vi "Initialize.vi"(5 "Replication Offset":dbl, 7 "Flip Rotation?":bool, 8 "error in (no error)":errorcluster, 9 "Spawner Early Search":T1, 10 "Initial Direction Offset":T1, 11 "Test in":refnum<class "Swarm.lvclass">) -> (0 "error out":errorcluster, 3 "Test out":refnum<class "Swarm.lvclass">)   [LabVIEW 2020, in "Swarm.lvclass"]
uses:
  Swarm.lvclass
  Type Defs/Direction Enum.ctl
  Type Defs/Action Enum.ctl
  Swarm.lvclass/Swarm.ctl
  Type Defs/SB Type Defs.lvlib
  Common/Common.lvlib
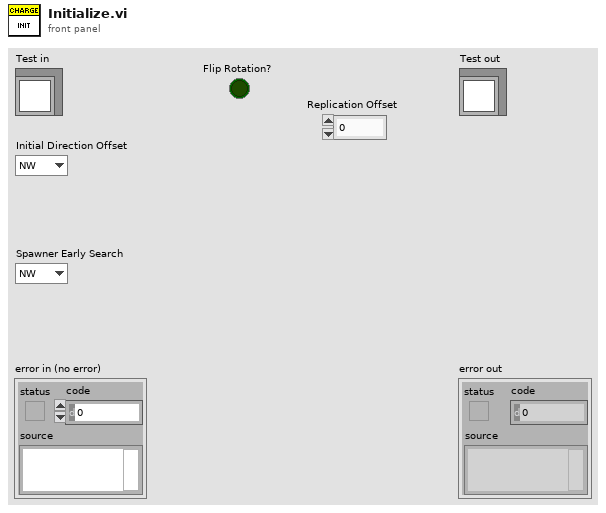
[diagram p1: front panel]
types:
  T1 = typedef "SB Type Defs.lvlib/Direction Enum.ctl" = enum16{"NW", "N", "NE", "E", "SE", "S", "SW", "W"}
  T2 = typedef "SB Type Defs.lvlib/Action Enum.ctl" = enum16{"Wait", "Move", "Attack", "Replicate"}
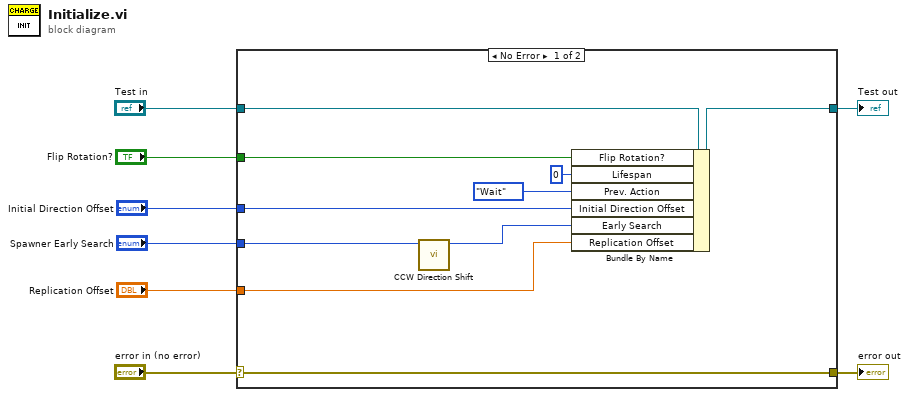
[diagram p0: block diagram]
diagram:
  n1 = case shown="No Error" "error in (no error)" {
    selector: "error in (no error)" -> [w18 w20]
    tunnel: [w18 w20] -> w7
    tunnel: [w15 w19] -> w5
    tunnel: "Test in" -> [w16 w19]
    tunnel: "Initial Direction Offset" -> [w14 _]
    tunnel: "Spawner Early Search" -> [w12 _]
    tunnel: "Flip Rotation?" -> [w10 _]
    tunnel: "Replication Offset" -> [w9 _]
    frame No Error {
      n2 = call "CCW Direction Shift.vi"("Direction"=w12) -> ("Numeric"=w11:i32)  [unwired: 10 in]
      n3 = Bundle By Name(cluster=w16, "Flip Rotation?"=w10, "Lifespan"=0, "Prev. Action"=Action_Enum."Wait", "Initial Direction Offset"=w14, "Early Search"=w11, "Replication Offset"=w9) -> (w15:refnum<class "Swarm.lvclass">)
    }
    frame Error {
    }
  }
  "error out" <- w7
  "Test out" <- w5
